vi "Stop Logging.vi"(8 "error in (no error)":errorcluster, 11 "Data Logger Interface in":refnum<class "TDMS Data Logger Actor.lvclass">) -> (0 "error out":errorcluster, 3 "Data Logger Interface out":refnum<class "TDMS Data Logger Actor.lvclass">)   [LabVIEW 2024, in "TDMS Data Logger Actor.lvlib" / "TDMS Data Logger Actor.lvclass"]
uses:
  TDMS Data Logger Actor.lvclass
  C:/Program Files (x86)/National Instruments/LabVIEW 2024/vi.lib/ActorFramework/Actor/Actor.lvclass
  TDMS Data Logger Actor.lvclass/TDMS Data Logger Actor.ctl
  <vilib>/ActorFramework/Actor/Actor.lvclass/Actor.ctl
  <vilib>/ActorFramework/Message Enqueuer/Message Enqueuer.lvclass/Message Enqueuer.ctl
  <vilib>/ActorFramework/Message Enqueuer/Enqueue.vi
  Data Logger Actor Reply Interface/Data Logger Actor Reply Interface Messages/Logging Stopped Msg/Logging Stopped Msg.lvclass
  C:/Program Files (x86)/National Instruments/LabVIEW 2024/vi.lib/ActorFramework/Message/Message.lvclass
  <vilib>/ActorFramework/Message Priority Queue/Priority Enqueue.vi
  <vilib>/ActorFramework/Actor/Actor.lvclass
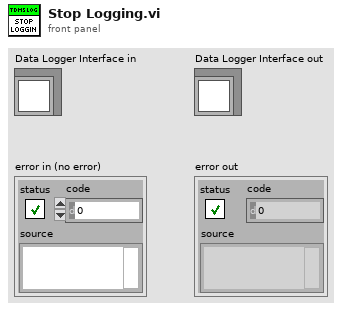
[diagram p1: front panel]
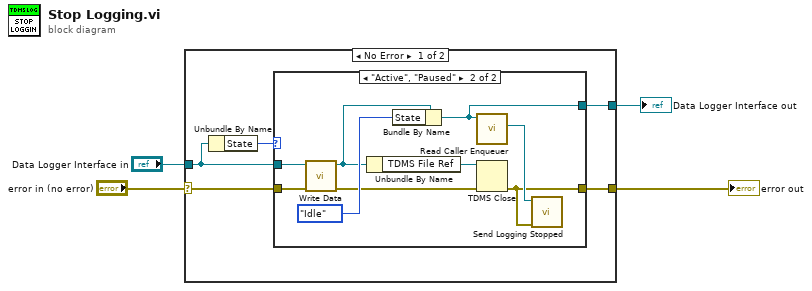
[diagram p0: block diagram]
diagram:
  n1 = case shown="No Error" "error in (no error)" {
    selector: "error in (no error)" -> [w7 w22]
    tunnel: "Data Logger Interface in" -> [w8 w21]
    tunnel: [w6 w22] -> w2
    tunnel: [w5 w21] -> w1
    frame No Error {
      n2 = Unbundle By Name(w8) -> ("State"=w9:enum16{"Idle", "Active", "Paused"})
      n3 = case shown="\"Active\", \"Paused\"" w9 {
        tunnel: w8 -> [w10 w16]
        tunnel: w7 -> [w11 w14]
        tunnel: [w11 w12] -> w6
        tunnel: [w10 w17] -> w5
        frame "Idle" {
        }
        frame "Active", "Paused" {
          n4 = call-dynamic "Write Data.vi"("error in (no error)"=w14, "TDMS Data Logger Actor in"=w16) -> ("error out"=w13:errorcluster, "TDMS Data Logger Actor out"=w15:refnum<class "TDMS Data Logger Actor.lvclass">)  [unwired: 8 in]
          n5 = Unbundle By Name(w15) -> ("TDMS File Ref"=w20:refnum<k34>)
          n6 = Bundle By Name(cluster=w15, "State"=enum16{"Idle", "Active", "Paused"}."Idle") -> (w17:refnum<class "TDMS Data Logger Actor.lvclass">)
          n7 = call <vilib>:"Read Caller Enqueuer.vi"("Actor"=w17) -> ("Caller Enqueuer"=w18:refnum<class "Message Enqueuer.lvclass">)  [unwired: 10 in]
          n8 = TDMS Close(8:w13, 11:w20) -> (0:w12:errorcluster)  [unwired: 1 out]
          n9 = call "Send Logging Stopped.vi"("error in (no error)"=w12, "Message Enqueuer"=w18) -> ()  [unwired: 8 in, 2 out]
        }
      }
    }
    frame Error {
    }
  }
  "error out" <- w2
  "Data Logger Interface out" <- w1
